vi "To XML.vi"(8 "error in (no error)":errorcluster, 11 "XMLInterface in":refnum<class "XmlInterface.lvclass">) -> (0 "error out":errorcluster, 2 "XML String":string, 3 "XMLInterface out":refnum<class "XmlInterface.lvclass">)   [LabVIEW 2027, in "XmlInterface.lvclass"]
uses:
  XmlInterface.lvclass
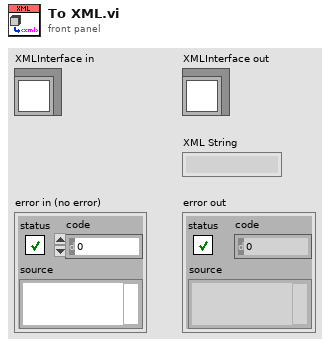
[diagram p1: front panel]
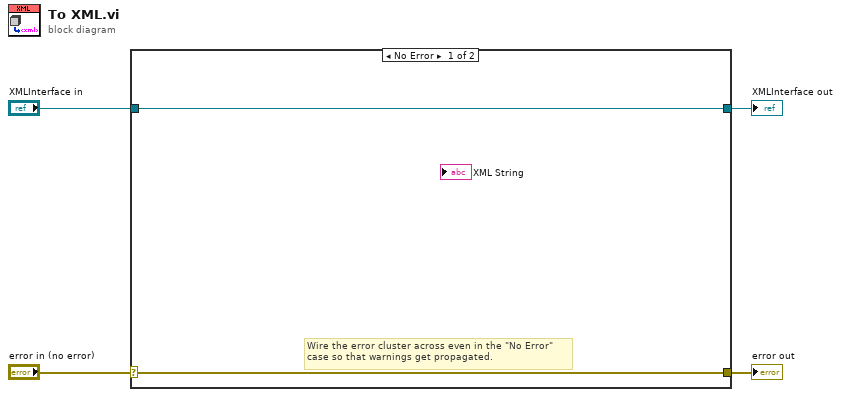
[diagram p0: block diagram]
diagram:
  n1 = case shown="No Error" "error in (no error)" {
    selector: "error in (no error)" -> [w6 w8]
    tunnel: [w6 w8] -> w3
    tunnel: [w5 w7] -> w1
    tunnel: "XMLInterface in" -> [w5 w7]
    frame No Error {
      # "Wire the error cluster across even in the \"No Error\"\ncase so that warnings get propagated."
    }
    frame Error {
    }
  }
  "error out" <- w3
  "XMLInterface out" <- w1
